vi "FT10_Fornax Check Power Level Correct.vi"(8 "Power Level in":T3, 9 "Mode in":T4, 10 "Port in":T5, 11 "JSON in":string) -> (2 "Valid?":T1=TRUE, 3 "Next Power Operation":T2)   [LabVIEW 2015]
uses:
  Controls/Control_Semi-Auto Port.ctl
  Controls/Control_Semi-Auto Mode.ctl
  Controls/Control_Semi-Auto Power Level.ctl
  Controls/Control_Auto - Next Power Operation.ctl
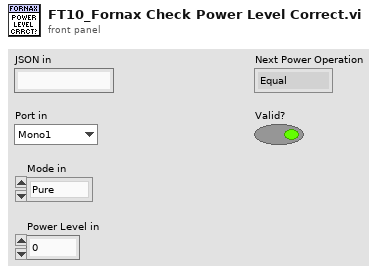
[diagram p1: front panel]
types:
  T1 = typedef "Control_Semi-Auto Power Level - Valid" = bool
  T2 = typedef "Control_Auto - Next Power Operation.ctl" = enum16{"Equal", "Power Down", "Power Up"}
  T3 = typedef "Control_Semi-Auto Power Level.ctl" = dbl
  T4 = typedef "Control_Semi-Auto Mode.ctl" = enum16{"Pure", "Blend", "Spray", "Fulgerate", "Standard", "Macro", "Precision", "Ligasure", "Error"}
  T5 = typedef "Control_Semi-Auto Port.ctl" = enum16{"Mono1", "Mono2", "Bipolar", "Ligasure", "Error"}
  T6 = typedef "Control_Fornax Bipolar Enum.ctl" = enum16{"Standard", "Macro", "Precision"}
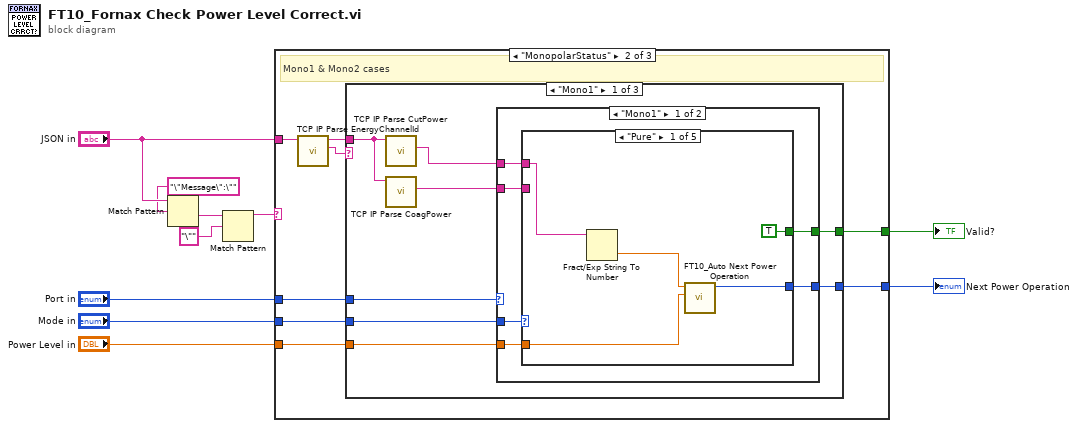
[diagram p0: block diagram]
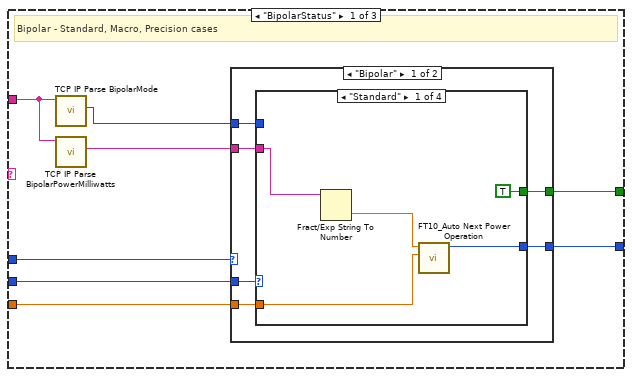
[diagram p2: hidden frame]
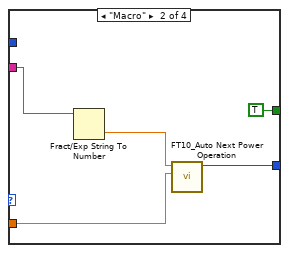
[diagram p3: hidden frame]
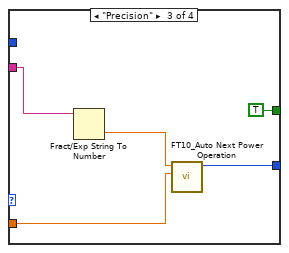
[diagram p4: hidden frame]
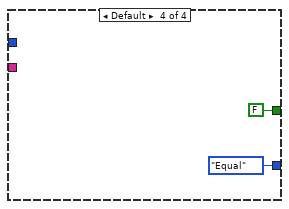
[diagram p5: hidden frame]
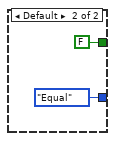
[diagram p6: hidden frame]
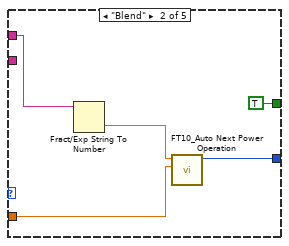
[diagram p7: hidden frame]
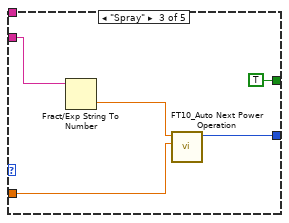
[diagram p8: hidden frame]
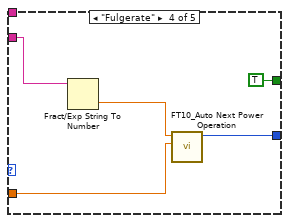
[diagram p9: hidden frame]
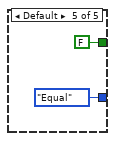
[diagram p10: hidden frame]
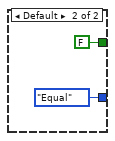
[diagram p11: hidden frame]
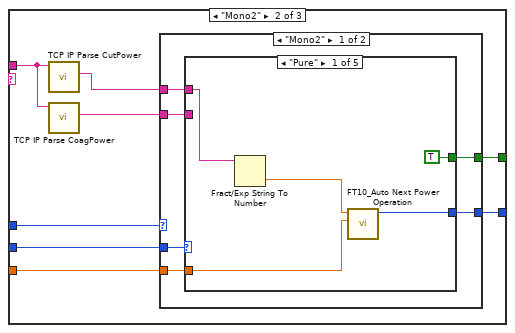
[diagram p12: hidden frame]
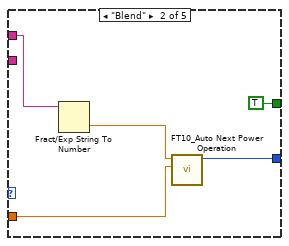
[diagram p13: hidden frame]
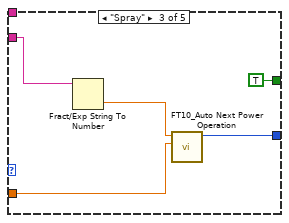
[diagram p14: hidden frame]
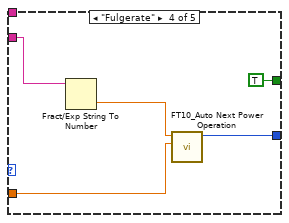
[diagram p15: hidden frame]
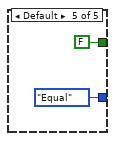
[diagram p16: hidden frame]
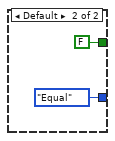
[diagram p17: hidden frame]
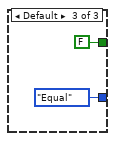
[diagram p18: hidden frame]
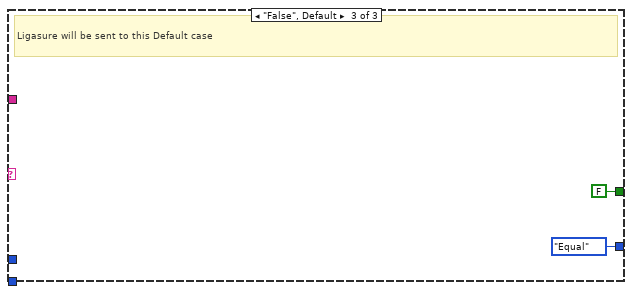
[diagram p19: hidden frame]
diagram:
  n1 = Match Pattern(string="JSON in", regular expression="\"Message\":\"") -> (after substring=w5:string)  [unwired: 1 in, 3 out]
  n2 = Match Pattern(string=w5, regular expression="\"") -> (before substring=w7:string)  [unwired: 1 in, 3 out]
  n3 = case shown="\"MonopolarStatus\"" w7 {
    tunnel: "JSON in" -> [w18 w51 _]
    tunnel: "Port in" -> [w17 w48 _]
    tunnel: "Mode in" -> [w16 w47 _]
    tunnel: "Power Level in" -> [w15 w46 _]
    tunnel: [w12 w45 T1 FALSE ("Valid?")] -> w2
    tunnel: [w11 w44 Control_Auto_-_Next_Power_Operation."Equal" ("Auto Tester - Next Power Operation")] -> w1
    frame "BipolarStatus" {
      # "Bipolar - Standard, Macro, Precision cases"
      n4 = call "TCP IP Parse BipolarMode.vi"("JSON in"=w18) -> ("Bipolar Enum"=w13:T6)  [unwired: 9 in, 1 out]
      n5 = call "TCP IP Parse BipolarPowerMilliwatts.vi"("JSON in"=w18) -> ("Bipolar Power (xx.x)"=w14:string)  [unwired: 9 in, 1 out]
      n6 = case shown="\"Bipolar\"" w17 {
        tunnel: w16 -> [w24 _]
        tunnel: w14 -> [w23 _]
        tunnel: w13 -> [w22 _]
        tunnel: w15 -> [w21 _]
        tunnel: [w20 T1 FALSE ("Valid?")] -> w12
        tunnel: [w19 Control_Auto_-_Next_Power_Operation."Equal" ("Auto Tester - Next Power Operation")] -> w11
        frame "Bipolar" {
          n7 = case shown="\"Standard\"" w24 {
            tunnel: w23 -> [w29 w34 w39 _]
            tunnel: w22 -> [_ _ _ _]
            tunnel: w21 -> [w27 w32 w37 _]
            tunnel: [T1 TRUE ("Valid?") T1 TRUE ("Valid?") T1 TRUE ("Valid?") T1 FALSE ("Valid?")] -> w20
            tunnel: [w26 w31 w36 Control_Auto_-_Next_Power_Operation."Equal" ("Auto Tester - Next Power Operation")] -> w19
            frame "Standard" {
              n8 = Fract/Exp String To Number(string=w29) -> (number=w25:dbl)  [unwired: 3 in, 1 out]
              n9 = call "FT10_Auto Next Power Operation.vi"("Power Level in"=w27, "Power Reading"=w25) -> ("Auto Tester - Next Power Operation"=w26:T2)  [unwired: 9 in]
            }
            frame "Macro" {
              n10 = Fract/Exp String To Number(string=w34) -> (number=w30:dbl)  [unwired: 3 in, 1 out]
              n11 = call "FT10_Auto Next Power Operation.vi"("Power Level in"=w32, "Power Reading"=w30) -> ("Auto Tester - Next Power Operation"=w31:T2)  [unwired: 9 in]
            }
            frame "Precision" {
              n12 = Fract/Exp String To Number(string=w39) -> (number=w35:dbl)  [unwired: 3 in, 1 out]
              n13 = call "FT10_Auto Next Power Operation.vi"("Power Level in"=w37, "Power Reading"=w35) -> ("Auto Tester - Next Power Operation"=w36:T2)  [unwired: 9 in]
            }
            frame Default {
            }
          }
        }
        frame Default {
        }
      }
    }
    frame "MonopolarStatus" {
      # "Mono1 & Mono2 cases"
      n14 = call "TCP IP Parse EnergyChannelId.vi"("JSON in"=w51) -> ("Energy Channel ID"=w49:string, "JSON out"=w50:string)  [unwired: 9 in]
      n15 = case shown="\"Mono1\"" w49 {
        tunnel: w50 -> [w59 w97 _]
        tunnel: w48 -> [w58 w94 _]
        tunnel: w47 -> [w57 w93 _]
        tunnel: w46 -> [w54 w92 _]
        tunnel: [w53 w91 T1 FALSE ("Valid?")] -> w45
        tunnel: [w52 w90 Control_Auto_-_Next_Power_Operation."Equal" ("Auto Tester - Next Power Operation")] -> w44
        frame "Mono1" {
          n16 = call "TCP IP Parse CutPower.vi"("JSON in"=w59) -> ("Cut Power"=w55:string)  [unwired: 9 in, 1 out]
          n17 = call "TCP IP Parse CoagPower.vi"("JSON in"=w59) -> ("Coag Power"=w56:string)  [unwired: 9 in, 1 out]
          n18 = case shown="\"Mono1\"" w58 {
            tunnel: w57 -> [w65 _]
            tunnel: w56 -> [w64 _]
            tunnel: w55 -> [w63 _]
            tunnel: w54 -> [w62 _]
            tunnel: [w61 T1 FALSE ("Valid?")] -> w53
            tunnel: [w60 Control_Auto_-_Next_Power_Operation."Equal" ("Auto Tester - Next Power Operation")] -> w52
            frame "Mono1" {
              n19 = case shown="\"Pure\"" w65 {
                tunnel: w64 -> [_ _ w80 w85 _]
                tunnel: w63 -> [w70 w75 _ _ _]
                tunnel: w62 -> [w68 w73 w78 w83 _]
                tunnel: [T1 TRUE ("Valid?") T1 TRUE ("Valid?") T1 TRUE ("Valid?") T1 TRUE ("Valid?") T1 FALSE ("Valid?")] -> w61
                tunnel: [w67 w72 w77 w82 Control_Auto_-_Next_Power_Operation."Equal" ("Auto Tester - Next Power Operation")] -> w60
                frame "Pure" {
                  n20 = Fract/Exp String To Number(string=w70) -> (number=w66:dbl)  [unwired: 3 in, 1 out]
                  n21 = call "FT10_Auto Next Power Operation.vi"("Power Level in"=w68, "Power Reading"=w66) -> ("Auto Tester - Next Power Operation"=w67:T2)  [unwired: 9 in]
                }
                frame "Blend" {
                  n22 = Fract/Exp String To Number(string=w75) -> (number=w71:dbl)  [unwired: 3 in, 1 out]
                  n23 = call "FT10_Auto Next Power Operation.vi"("Power Level in"=w73, "Power Reading"=w71) -> ("Auto Tester - Next Power Operation"=w72:T2)  [unwired: 9 in]
                }
                frame "Spray" {
                  n24 = Fract/Exp String To Number(string=w80) -> (number=w76:dbl)  [unwired: 3 in, 1 out]
                  n25 = call "FT10_Auto Next Power Operation.vi"("Power Level in"=w78, "Power Reading"=w76) -> ("Auto Tester - Next Power Operation"=w77:T2)  [unwired: 9 in]
                }
                frame "Fulgerate" {
                  n26 = Fract/Exp String To Number(string=w85) -> (number=w81:dbl)  [unwired: 3 in, 1 out]
                  n27 = call "FT10_Auto Next Power Operation.vi"("Power Level in"=w83, "Power Reading"=w81) -> ("Auto Tester - Next Power Operation"=w82:T2)  [unwired: 9 in]
                }
                frame Default {
                }
              }
            }
            frame Default {
            }
          }
        }
        frame "Mono2" {
          n28 = call "TCP IP Parse CutPower.vi"("JSON in"=w97) -> ("Cut Power"=w96:string)  [unwired: 9 in, 1 out]
          n29 = call "TCP IP Parse CoagPower.vi"("JSON in"=w97) -> ("Coag Power"=w95:string)  [unwired: 9 in, 1 out]
          n30 = case shown="\"Mono2\"" w94 {
            tunnel: w93 -> [w103 _]
            tunnel: w95 -> [w102 _]
            tunnel: w96 -> [w101 _]
            tunnel: w92 -> [w100 _]
            tunnel: [w99 T1 FALSE ("Valid?")] -> w91
            tunnel: [w98 Control_Auto_-_Next_Power_Operation."Equal" ("Auto Tester - Next Power Operation")] -> w90
            frame "Mono2" {
              n31 = case shown="\"Pure\"" w103 {
                tunnel: w102 -> [_ _ w118 w123 _]
                tunnel: w101 -> [w108 w113 _ _ _]
                tunnel: w100 -> [w105 w110 w116 w121 _]
                tunnel: [T1 TRUE ("Valid?") T1 TRUE ("Valid?") T1 TRUE ("Valid?") T1 TRUE ("Valid?") T1 FALSE ("Valid?")] -> w99
                tunnel: [w106 w111 w115 w120 Control_Auto_-_Next_Power_Operation."Equal" ("Auto Tester - Next Power Operation")] -> w98
                frame "Pure" {
                  n32 = Fract/Exp String To Number(string=w108) -> (number=w104:dbl)  [unwired: 3 in, 1 out]
                  n33 = call "FT10_Auto Next Power Operation.vi"("Power Level in"=w105, "Power Reading"=w104) -> ("Auto Tester - Next Power Operation"=w106:T2)  [unwired: 9 in]
                }
                frame "Blend" {
                  n34 = Fract/Exp String To Number(string=w113) -> (number=w109:dbl)  [unwired: 3 in, 1 out]
                  n35 = call "FT10_Auto Next Power Operation.vi"("Power Level in"=w110, "Power Reading"=w109) -> ("Auto Tester - Next Power Operation"=w111:T2)  [unwired: 9 in]
                }
                frame "Spray" {
                  n36 = Fract/Exp String To Number(string=w118) -> (number=w114:dbl)  [unwired: 3 in, 1 out]
                  n37 = call "FT10_Auto Next Power Operation.vi"("Power Level in"=w116, "Power Reading"=w114) -> ("Auto Tester - Next Power Operation"=w115:T2)  [unwired: 9 in]
                }
                frame "Fulgerate" {
                  n38 = Fract/Exp String To Number(string=w123) -> (number=w119:dbl)  [unwired: 3 in, 1 out]
                  n39 = call "FT10_Auto Next Power Operation.vi"("Power Level in"=w121, "Power Reading"=w119) -> ("Auto Tester - Next Power Operation"=w120:T2)  [unwired: 9 in]
                }
                frame Default {
                }
              }
            }
            frame Default {
            }
          }
        }
        frame Default {
        }
      }
    }
    frame "False", Default {
      # "Ligasure will be sent to this Default case"
    }
  }
  "Next Power Operation" <- w1
  "Valid?" <- w2
